vi "XY Graph Show-Hide Tool Panels Event.vi"(8 "Error In":errorcluster, 11 "XYGraph in":T1) -> (0 "Error Out":errorcluster, 1 "Message":string, 3 "Tool Panels Shown?":bool)   [LabVIEW 2021, in "XY Graph Add-Ons.lvlib"]
uses:
  XY Graph Add-Ons.lvlib
  XY Graph Refnum.ctl
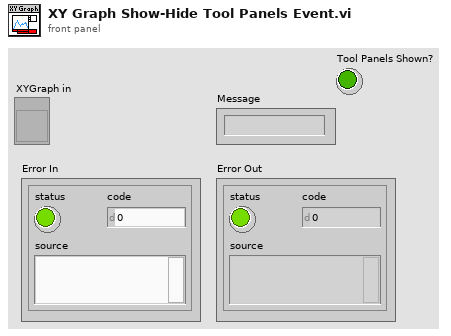
[diagram p1: front panel]
types:
  T1 = typedef "XY Graph Add-Ons.lvlib/XY Graph Refnum.ctl" = refnum<vi>
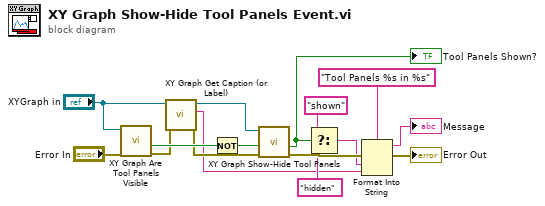
[diagram p0: block diagram]
diagram:
  n1 = call "XY Graph Are Tool Panels Visible.vi"("Error In"="Error In", "XY Graph Ref"="XYGraph in") -> ("Error Out"=w3:errorcluster, "Any Panel Visible?"=w6:bool)  [unwired: 6 in, 2 out]
  n2 = call "XY Graph Get Caption (or Label).vi"("error in (no error)"=w3, "XYGraph in"="XYGraph in") -> ("error out"=w2:errorcluster, "Caption (or Label) Text"=w1:string, "XYGraph out"=w4:T1)  [unwired: 7 in]
  n3 = Not(x=w6) -> (.not. x?=w5:bool)
  n4 = call "XY Graph Show-Hide Tool Panels.vi"("Error In"=w2, "Hide (F) /Show (T)"=w5, "XY Graph Ref"=w4) -> ("Error Out"=w16:errorcluster, "Tool Panels Shown?"=w12:bool)  [unwired: 7 in]
  "Tool Panels Shown?" <- w12
  n5 = Select(t="shown" ("format string"), s=w12, f="hidden" ("format string")) -> (s? t:f=w9:string)
  n6 = Format Into String(format string="Tool Panels %s in %s", error in=w16, w9, w1) -> (resulting string=→"Message":string, error out=→"Error Out":errorcluster)  [unwired: 1 in]
